vi "GUI Queue Handler.vi"(7 "Action":T3, 8 "error in (no error)":errorcluster, 10 "Message in":T1, 11 "User event in":refnum<user-event>) -> (0 "error out":errorcluster, 1 "Event Registration Refnum":refnum<event-registration>, 2 "Timeout":i32, 3 "User event out":refnum<user-event>)   [LabVIEW 2017]
uses:
  Type Definitions/Queue FG Options.ctl
  Type Definitions/GUI Message.ctl
  Type Definitions/Controller States.ctl
  Type Definitions/Timer States.ctl
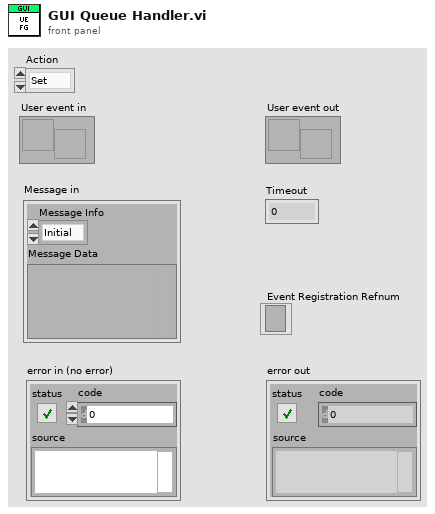
[diagram p1: front panel]
types:
  T1 = typedef "GUI Message.ctl" = cluster{"Message Info":T2, "Message Data":variant}
  T2 = typedef "Controller States.ctl" = enum16{"Initial", "Login", "Idle", "Balance Inquiry", "Deposit", "Withdrawal", "Fast Cash", "Terminate", "Shutdown"}
  T3 = typedef "Queue FG Options.ctl" = enum16{"Set", "Get", "Read", "Write", "Destroy"}
  T4 = typedef "Timer States.ctl" = enum16{"Set", "Get"}
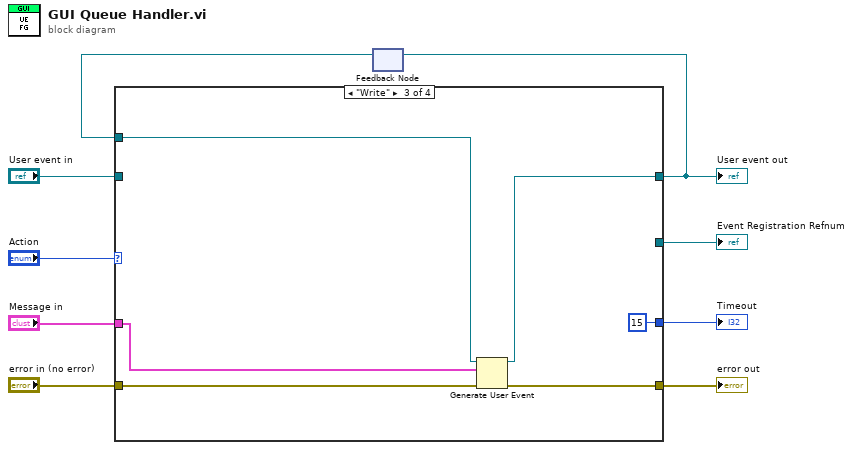
[diagram p0: block diagram]
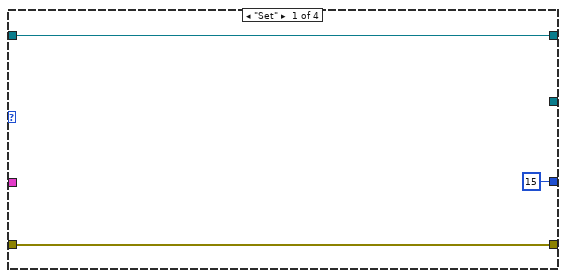
[diagram p2: hidden frame]
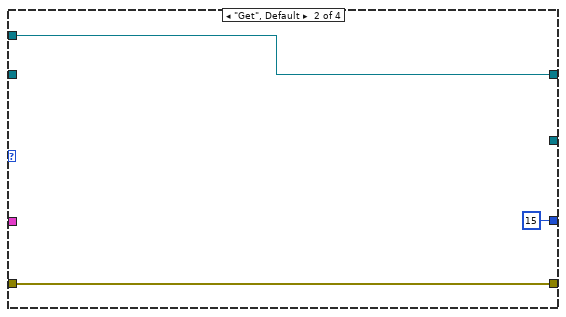
[diagram p3: hidden frame]
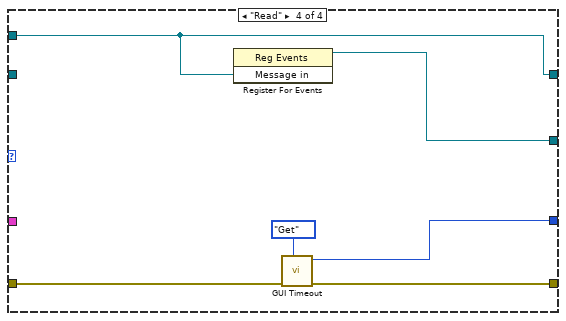
[diagram p4: hidden frame]
diagram:
  n1 = feedback #1() -> (w6:refnum<user-event>)  [unwired: 1 in]
  n2 = case shown="\"Write\"" "Action" {
    tunnel: "error in (no error)" -> [w12 w15 w21 w27]
    tunnel: [w12 w15 w20 w25] -> w7
    tunnel: w6 -> [_ w13 w17 w22]
    tunnel: "Message in" -> [_ _ w16 _]
    tunnel: [_ _ _ w26] -> w1
    tunnel: [15 ("Timeout") 15 ("Timeout") 15 ("Timeout") w23] -> w4
    tunnel: [w10 w13 w18 w22] -> w3
    tunnel: "User event in" -> [w10 _ _ _]
    frame "Set" {
    }
    frame "Get", Default {
    }
    frame "Write" {
      n3 = Generate User Event(user event=w17, event data cluster=w16, error in=w21) -> (user event out=w18:refnum<user-event>, error out=w20:errorcluster)  [unwired: 1 in]
    }
    frame "Read" {
      n4 = register-events(w22) -> (reference out=w26:refnum<event-registration>)  [unwired: 2 in, 1 out]
      n5 = call "GUI Timeout.vi"("Timer States"=Timer_States."Get", "error in (no error)"=w27) -> ("error out"=w25:errorcluster, "Timeout"=w23:i32)  [unwired: 8 in]
    }
  }
  "error out" <- w7
  "Timeout" <- w4
  "User event out" <- w3
  "Event Registration Refnum" <- w1
  n6 = feedback-in #1(w3) -> ()
